vi "Teleop.vi"(10 "Match Info":T1={"Autonomous Elapsed Seconds"=0.0, "TeleOp Elapsed Seconds"=0.0, "Disabled Elapsed Seconds"=0.0, "Visited Autonomous"=FALSE, "Visited TeleOp"=FALSE, "Visited Disabled"=FALSE, "Autonomous Settings"={"Autonomous Style"=enum."Independent", "VI Refnum"=refnum}}, 11 "Call Context":T2) -> ()   [LabVIEW 2013]
doc: "This VI is called for each TeleOp packet received from the DS where the robot is not disabled. It is often used to read from the joysticks and update I/O or to update setpoints for timed control loops. It should complete and return within 20 milliseconds or it may miss DS packets."
uses:
  <vilib>/Rock Robotics/WPI/DriverStation/WPI_DriverStationDerivedRobotMode.ctl
  <vilib>/Rock Robotics/WPI/DriverStation/WPI_DriverStationMatch Info.ctl
  <vilib>/Rock Robotics/WPI/DriverStation/DriverStationLCD/WPI_DriverStationLCDLCDLine.ctl
  Robot Global Data.vi
  <vilib>/Rock Robotics/WPI/Joystick/WPI_JoystickGetSetRefNum.vi
  <vilib>/Rock Robotics/WPI/RobotDrive/WPI_RobotDriveGetSetRefNum.vi
  <vilib>/Rock Robotics/WPI/Solenoid/WPI_SolenoidSetEnum.vi
  <vilib>/Rock Robotics/WPI/Solenoid/WPI_SolenoidValue.ctl
panel:
  out "Numeric 1":dbl(slide) scale=0.0..100.0
  out "Boolean 2":bool
  out "Boolean 1":bool
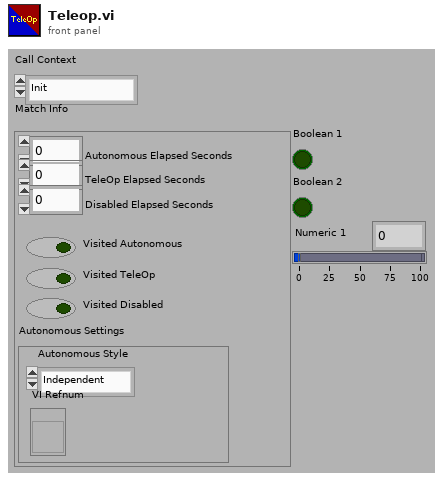
[diagram p1: front panel]
types:
  T1 = typedef "WPI_DriverStationMatch Info.ctl" = cluster{"Autonomous Elapsed Seconds":dbl, "TeleOp Elapsed Seconds":dbl, "Disabled Elapsed Seconds":dbl, "Visited Autonomous":bool, "Visited TeleOp":bool, "Visited Disabled":bool, "Autonomous Settings":cluster{"Autonomous Style":enum16{"Iterative", "Independent"}, "VI Refnum":refnum<vi>}}
  T2 = typedef "WPI_DriverStationDerivedRobotMode.ctl" = enum16{"Init", "Execute", "Stop"}
  T3 = typedef "WPI_DriverStationLCDLCDLine.ctl" = enum16{"Main - Line 1", "User - Line 2", "User - Line 3", "User - Line 4", "User - Line 5", "User - Line 6"}
  T4 = typedef "WPI_JoystickDevRef.ctl" = cluster{"Device":T5}
  T5 = typedef "WPI_JoystickDeviceEnum.ctl" = enum16{"USB 1", "USB 2", "USB 3", "USB 4", "Kinect 1", "Kinect 2"}
  T6 = typedef "WPI_JoystickButtonState.ctl" = cluster{"Button 1":bool, "Button 2":bool, "Button 3":bool, "Button 4":bool, "Button 5":bool, "Button 6":bool, "Button 7":bool, "Button 8":bool, "Button 9":bool, "Button 10":bool, "Button 11":bool, "Button 12":bool}
  T7 = cluster{"axis 1 (x)":dbl, "axis 2 (y)":dbl, "axis 3 (throttle)":dbl, "axis 4":dbl, "axis 5":dbl, "axis 6":dbl}
  T8 = typedef "WPI_SolenoidValue.ctl" = enum16{"Off", "On", "Forward", "Reverse"}
  T9 = typedef "WPI_SolenoidDevRef.ctl" = cluster{"DevStatus":errorcluster, "Solenoid Module":T10, "Forward Solenoid Channel":T11, "Reverse Solenoid Channel":T11}
  T10 = typedef "FPGA_TypedefSolenoidModule.ctl" = enum16{"Solenoid Module 1", "Solenoid Module 2"}
  T11 = typedef "WPI_SolenoidChannel.ctl" = enum8{"Solenoid 1", "Solenoid 2", "Solenoid 3", "Solenoid 4", "Solenoid 5", "Solenoid 6", "Solenoid 7", "Solenoid 8", "Invalid"}
  T12 = typedef "WPI_RobotDriveDevRef.ctl" = cluster{"DevStatus":errorcluster, "Motors[]":T13[], "Square Inputs":bool, "Max Output":dbl, "Isochronous":bool}
  T13 = typedef "WPI_MotorControlDeviceRef.ctl" = cluster{"DeviceStatus":errorcluster, "Type":enum16{"PWM", "CAN"}, "PWM":cluster{"Digital Module":T14, "PWM Channel":T15, "DeadBand":T16}, "CAN":cluster{"Device Number":u8, "Control Mode":T17, "Semaphore":T18, "Max Vout":dbl}, "Invert":bool, "TransformRef":T19, "InvTransformRef":T19}
  T14 = typedef "FPGA_TypedefDigitalModule.ctl" = enum16{"Digital Module 1", "Digital Module 2"}
  T15 = typedef "FPGA_DIOPWMChannel.ctl" = enum8{"PWM 1", "PWM 2", "PWM 3", "PWM 4", "PWM 5", "PWM 6", "PWM 7", "PWM 8", "PWM 9", "PWM 10", "Invalid"}
  T16 = typedef "WPI_PWMDeadband.ctl" = cluster{"Name":string, "maxPositivePwm":i32, "minPositivePwm":i32, "centerPwm":i32, "maxNegativePwm":i32, "minNegativePwm":i32, "angularRange":u16}
  T17 = typedef "WPI_CANJaguar_ControlMode.ctl" = enum8{"Percent VBus", "Current", "Speed", "Position", "Voltage"}
  T18 = typedef "Semaphore RefNum" = refnum<k1>
  T19 = typedef "WPI_PWMTransform_ConPane.ctl" = refnum<vi>
  T20 = enum16{"Reset", "Start", "Reset 2", "Manual", "Get ready to Fire", "Disengage Gearbox", "Ready to Fire", "Firing", "Firing Completed", "Reengage Gearbox"}
  T21 = typedef "WPI_DigitalInputDevRef.ctl" = cluster{"DevStatus":errorcluster, "DIO Channel":T22, "Digital Module":T14}
  T22 = typedef "FPGA_DIOChannel.ctl" = enum8{"DIO 1", "DIO 2", "DIO 3", "DIO 4", "DIO 5", "DIO 6", "DIO 7", "DIO 8", "DIO 9", "DIO 10", "DIO 11", "DIO 12", "DIO 13", "DIO 14", "Invalid"}
  T23 = typedef "WPI_AnalogChannelDevRef.ctl" = cluster{"DevStatus":errorcluster, "Analog Module":T24, "Analog Channel":T25}
  T24 = typedef "FPGA_TypedefAnalogModule.ctl" = enum16{"Analog Module 1", "Analog Module 2"}
  T25 = typedef "FPGA_AIChannel.ctl" = enum8{"AI 1", "AI 2", "AI 3", "AI 4", "AI 5", "AI 6", "AI 7", "AI 8", "Invalid"}
  T26 = typedef "WPI_RelayDevRef.ctl" = cluster{"DevStatus":errorcluster, "Relay Channel":T27, "Digital Module":T14, "Relay Direction":T28}
  T27 = typedef "FPGA_DIORelayChannel.ctl" = enum8{"Relay 1", "Relay 2", "Relay 3", "Relay 4", "Relay 5", "Relay 6", "Relay 7", "Relay 8", "Invalid"}
  T28 = typedef "WPI_RelayDirection.ctl" = enum16{"Both directions", "Forward only", "Reverse only"}
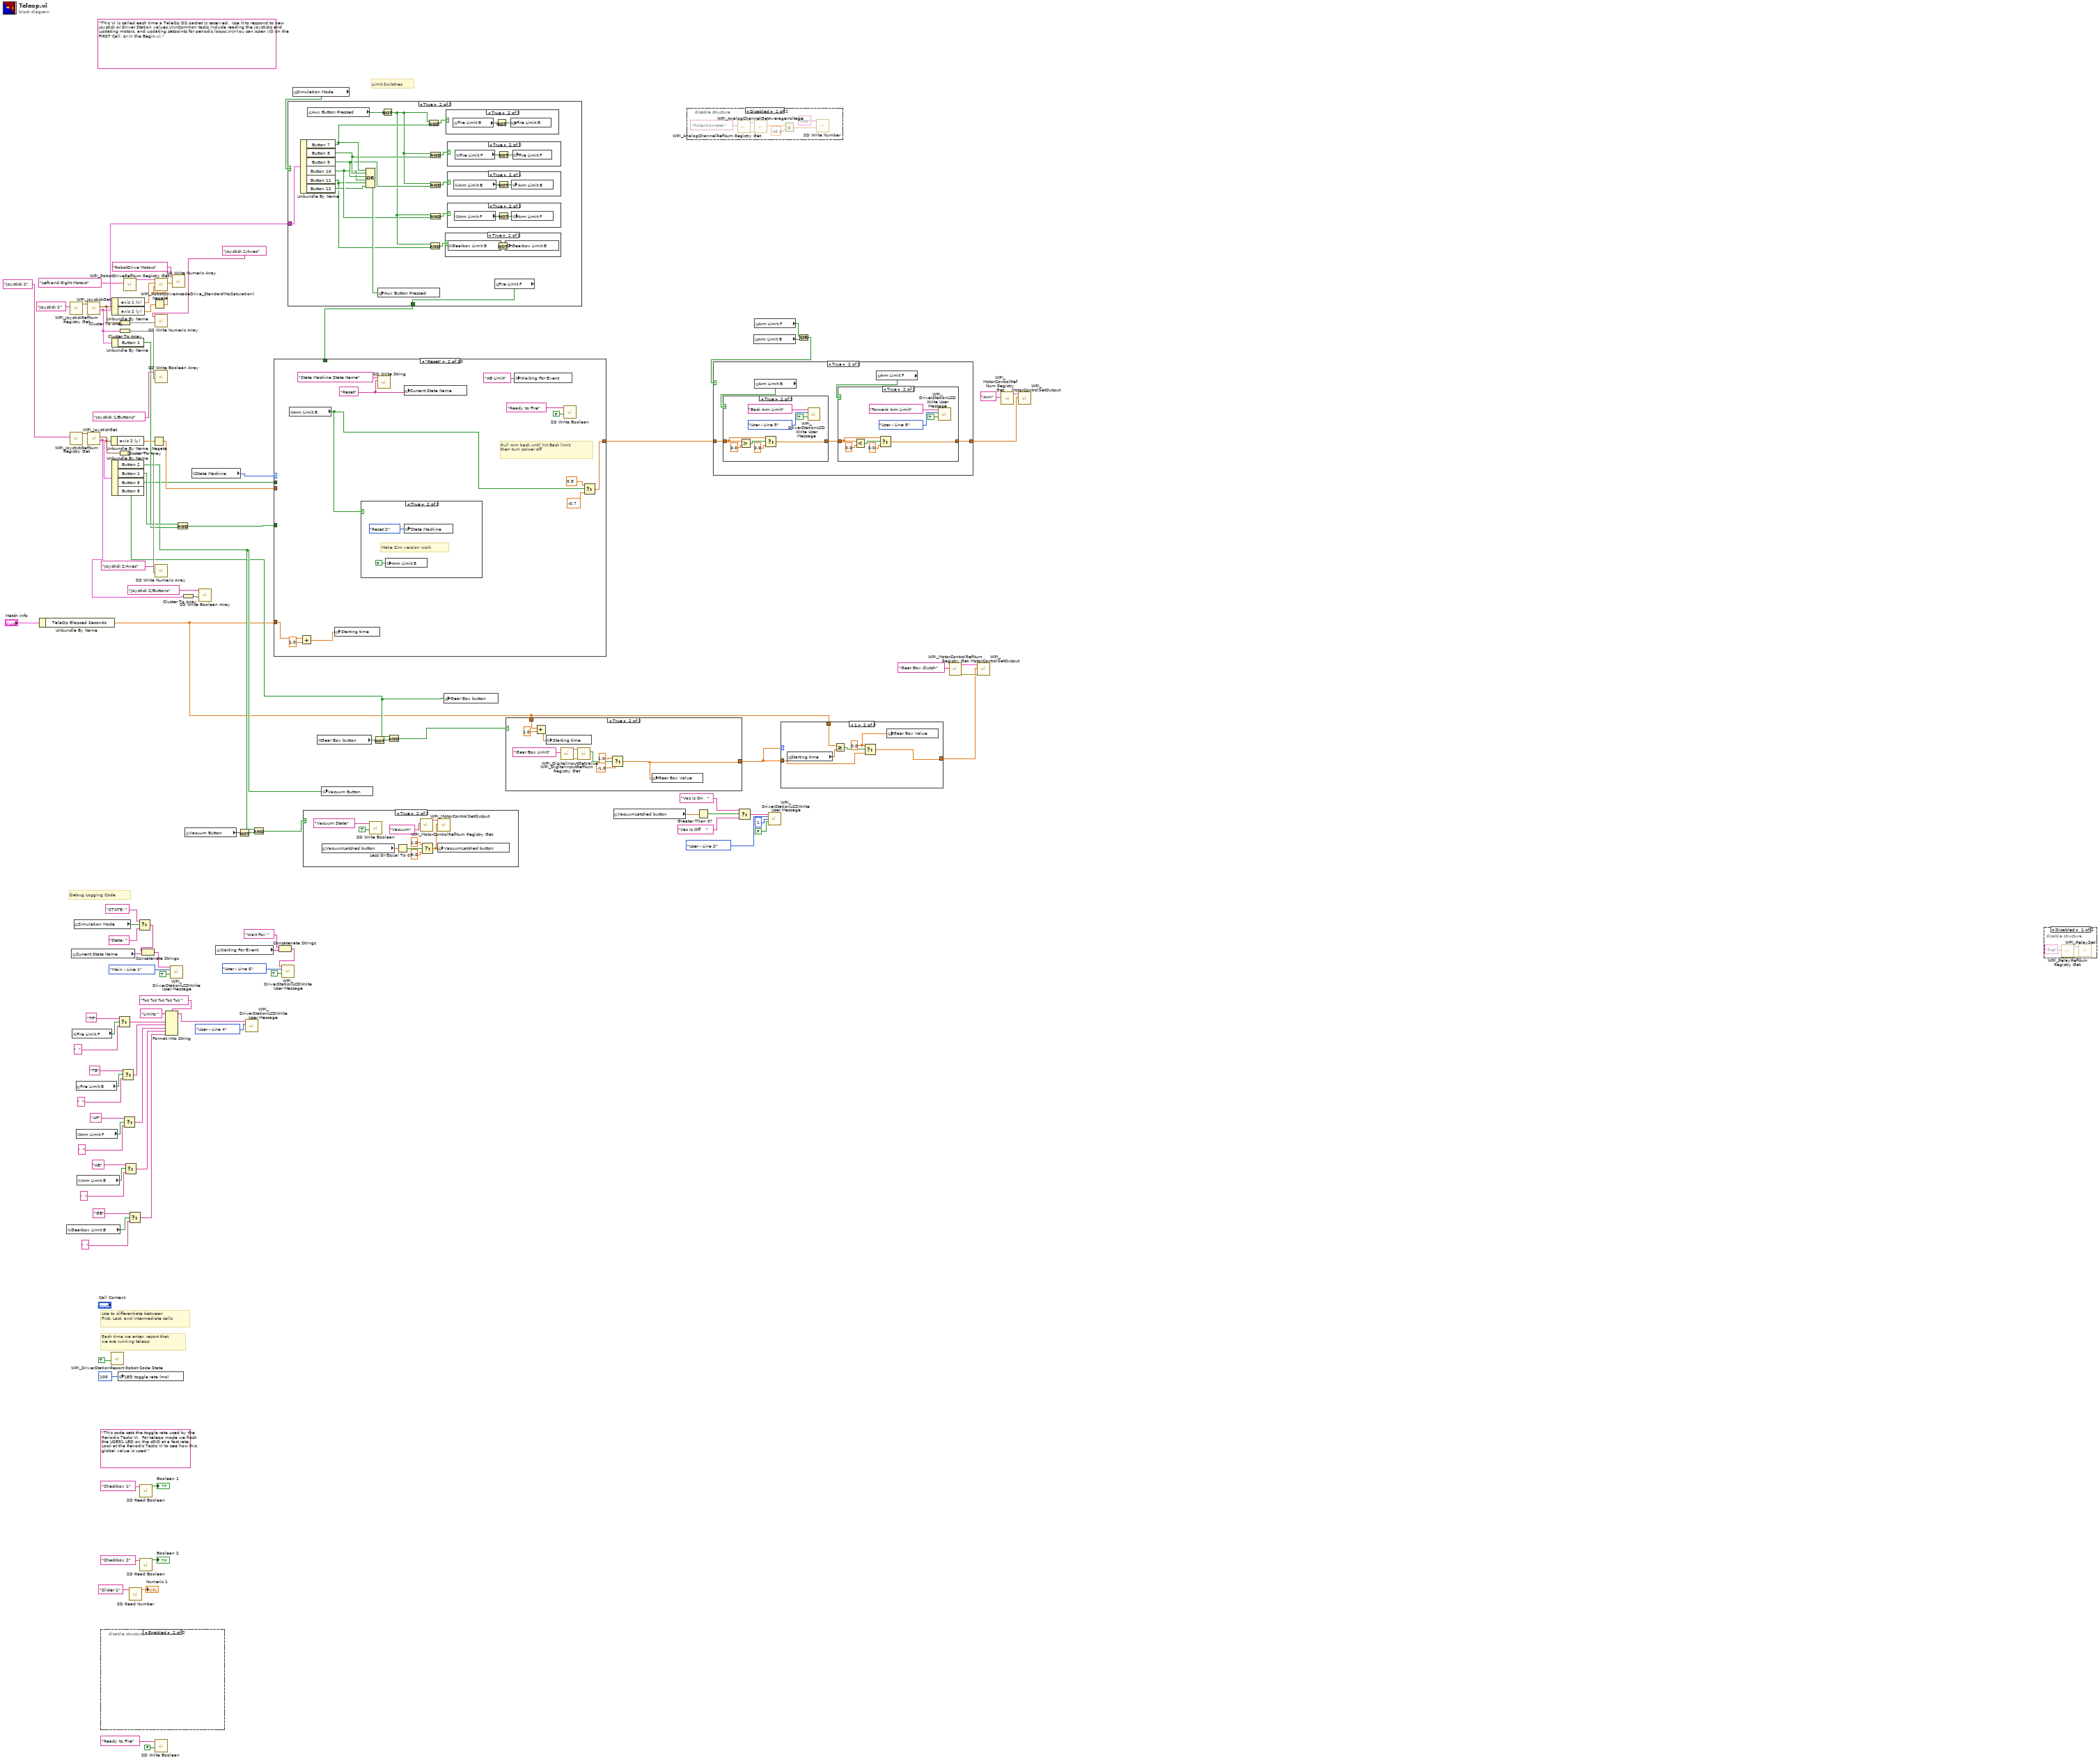
[diagram p0: block diagram]
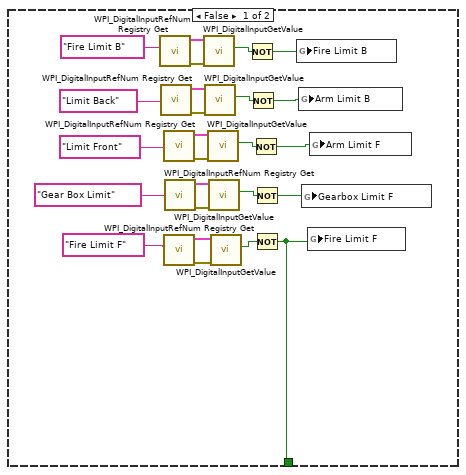
[diagram p2: hidden frame]
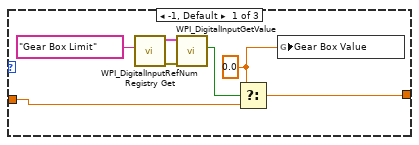
[diagram p8: hidden frame]
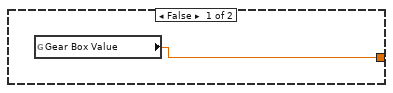
[diagram p10: hidden frame]
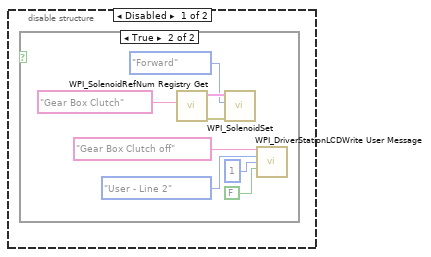
[diagram p17: hidden frame]
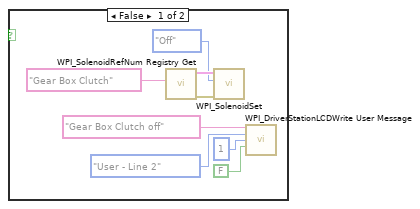
[diagram p18: hidden frame]
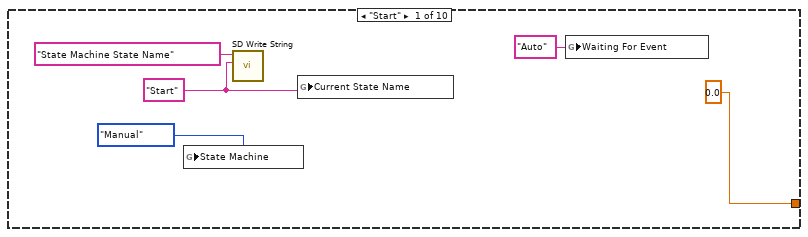
[diagram p19: hidden frame]
diagram:
  (unwired) "This code sets the toggle rate used by the Periodic Tasks VI.  For teleop mode we flash the USER1 LED on the cRIO at a fast rate.  Look at the Periodic Tasks VI to see how this global value is used."
  (unwired) "This VI is called each time a TeleOp DS packet is received.  Use it to respond to new joystick or Driver Station values.\n\nCommon tasks include reading the joysticks and updating motors, and updating setpoints for periodic loops.\n\nYou can open I/O on the FIRST Call, or in the Begin.vi."
  # "Limit Switches"
  # "Debug Logging Code"
  # "Each time we enter, report that\nwe are running teleop"
  # "Use to differentiate between\nFirst, Last, and Intermediate calls"
  n1 = Unbundle By Name("Match Info") -> ("TeleOp Elapsed Seconds"=w36:dbl)
  n2 = global read "Robot Global Data.vi" "Gearbox Limit B"() -> (w17:bool)
  n3 = call <vilib>:"WPI_JoystickRefNum Registry Get.vi"("refnum name"="Joystick 1") -> ("JoystickDevRef"=w104:T4)  [unwired: 1 in, 9 out]
  n4 = call <vilib>:"WPI_JoystickRefNum Registry Get.vi"("refnum name"="Joystick 2") -> ("JoystickDevRef"=w87:T4)  [unwired: 1 in, 9 out]
  n5 = global read "Robot Global Data.vi" "Current State Name"() -> (w52:string)
  n6 = global read "Robot Global Data.vi" "Fire Limit F"() -> (w21:bool)
  n7 = global read "Robot Global Data.vi" "Simulation Mode"() -> (w10:bool)
  n8 = global read "Robot Global Data.vi" "Fire Limit B"() -> (w20:bool)
  n9 = global read "Robot Global Data.vi" "Arm Limit F"() -> (w19:bool)
  n10 = global read "Robot Global Data.vi" "Arm Limit B"() -> (w18:bool)
  n11 = call <vilib>:"WPI_JoystickGet.vi"("JoystickDevRef"=w104) -> ("Buttons"=w6:T6, "Axes"=w99:T7)  [unwired: 1 in, 4 out]
  n12 = call <vilib>:"WPI_JoystickGet.vi"("JoystickDevRef"=w87) -> ("Buttons"=w81:T6, "Axes"=w84:T7)  [unwired: 1 in, 4 out]
  n13 = disable-structure shown="Enabled" {
    frame Disabled {
      n14 = case shown="True" {
        selector: _ -> [_ _]
        frame False {
          n15 = call <vilib>:"WPI_SolenoidRefNum Registry Get.vi"("refnum name"="Gear Box Clutch") -> ("error out"=w115:errorcluster, "SolenoidDevRef"=w116:T9)  [unwired: 9 in]
          n16 = call-poly <vilib>:"WPI_SolenoidSet.vi"("error in (no error)"=w115, "Value"=WPI_SolenoidValue."Off", "SolenoidDevRef"=w116) -> ()  [unwired: 7 in, 2 out]
          n17 = call <vilib>:"WPI_DriverStationLCDWrite User Message.vi"("line text"="Gear Box Clutch off", "line"=WPI_DriverStationLCDLCDLine."User - Line 2", "starting column"=i8 1, "clear line before write (T)"=FALSE) -> ()  [unwired: 11 in, 1 out]
        }
        frame True {
          n18 = call <vilib>:"WPI_SolenoidRefNum Registry Get.vi"("refnum name"="Gear Box Clutch") -> ("error out"=w123:errorcluster, "SolenoidDevRef"=w124:T9)  [unwired: 9 in]
          n19 = call-poly <vilib>:"WPI_SolenoidSet.vi"("error in (no error)"=w123, "Value"=WPI_SolenoidValue."Forward", "SolenoidDevRef"=w124) -> ()  [unwired: 7 in, 2 out]
          n20 = call <vilib>:"WPI_DriverStationLCDWrite User Message.vi"("line text"="Gear Box Clutch off", "line"=WPI_DriverStationLCDLCDLine."User - Line 2", "starting column"=i8 1, "clear line before write (T)"=FALSE) -> ()  [unwired: 11 in, 1 out]
        }
      }
    }
    frame Enabled {
    }
  }
  n21 = Unbundle By Name(w84) -> ("axis 2 (y)"=w80:dbl)
  n22 = call <vilib>:"WPI_DriverStationReport Robot Code State.vi"("TeleOp"=TRUE ("Autonomous")) -> ()  [unwired: 10 in, 1 out]
  n23 = Unbundle By Name(w99) -> ("axis 1 (x)"=w106:dbl, "axis 2 (y)"=w47:dbl)
  n24 = Unbundle By Name(w6) -> ("Button 1"=w78:bool)
  n25 = Unbundle By Name(w81) -> ("Button 2"=w69:bool, "Button 1"=w79:bool, "Button 5"=w55:bool, "Button 8"=w39:bool)
  n26 = Select(t="TF", s=w21, f="  ") -> (s? t:f=w27:string)
  n27 = global write "Robot Global Data.vi" "LED toggle rate (ms)"(u32 100 ("LED ms toggle rate")) -> ()
  n28 = Cluster To Array(cluster=w99) -> (array=w98:dbl[])
  n29 = Cluster To Array(cluster=w6) -> (array=w101:bool[])
  n30 = Cluster To Array(cluster=w84) -> (array=w83:dbl[])
  n31 = Select(t="TB", s=w20, f="  ") -> (s? t:f=w26:string)
  n32 = Select(t="AF", s=w19, f="  ") -> (s? t:f=w25:string)
  n33 = call <vilib>:"WPI_RobotDriveRefNum Registry Get.vi"("refnum name"="Left and Right Motors") -> ("RobotDriveDevRef"=w107:T12)  [unwired: 1 in, 9 out]
  n34 = Select(t="AB", s=w18, f="  ") -> (s? t:f=w24:string)
  n35 = Select(t="GB", s=w17, f="  ") -> (s? t:f=w23:string)
  n36 = call <vilib>:"SD Read Number.vi"("Name"="Slider 1" ("refnum name")) -> ("Numeric"=→"Numeric 1":dbl)  [unwired: 8 in, 2 out]
  n37 = Select(t="STATE: " ("line text"), s=w10, f="State: " ("line text")) -> (s? t:f=w7:string)
  n38 = call <vilib>:"SD Read Boolean.vi"("Name"="Checkbox 1" ("refnum name")) -> ("Boolean"=→"Boolean 1":bool)  [unwired: 8 in, 2 out]
  n39 = call <vilib>:"SD Read Boolean.vi"("Name"="Checkbox 2" ("refnum name")) -> ("Boolean"=→"Boolean 2":bool)  [unwired: 8 in, 2 out]
  n40 = Concatenate Strings(w7, w52) -> (w51:string)
  n41 = Negate(x=w80) -> (-x=w72:dbl)
  n42 = Negate(x=w47) -> (-x=w46:dbl)
  n43 = call <vilib>:"SD Write Boolean.vi"("Boolean"=FALSE, "Name"="Ready to Fire") -> ()  [unwired: 8 in, 2 out]
  n44 = call <vilib>:"WPI_RobotDriveArcadeDrive_Standard(NoSaturation).vi"("Y axis value"=w46, "X axis value"=w106, "RobotDriveDevRef"=w107) -> ("Motor Values"=w95:dbl[])  [unwired: 1 in, 7 out]
  n45 = call <vilib>:"SD Write Numeric Array.vi"("Numeric Array"=w98, "Name"="Joystick 1/Axes") -> ()  [unwired: 8 in, 2 out]
  n46 = call <vilib>:"SD Write Boolean Array.vi"("Boolean Array"=w101, "Name"="Joystick 1/Buttons") -> ()  [unwired: 8 in, 2 out]
  n47 = call <vilib>:"SD Write Numeric Array.vi"("Numeric Array"=w83, "Name"="Joystick 2/Axes") -> ()  [unwired: 8 in, 2 out]
  n48 = Format Into String(format string="%s %s %s %s %s " ("initial string"), initial string="Limits ", w27, w26, w25, w24, w23) -> (resulting string=w22:string)  [unwired: 1 in, 1 out]
  n49 = call <vilib>:"WPI_DriverStationLCDWrite User Message.vi"("line text"=w51, "line"=WPI_DriverStationLCDLCDLine."Main - Line 1", "clear line before write (T)"=TRUE) -> ()  [unwired: 12 in, 1 out]
  n50 = call <vilib>:"SD Write Numeric Array.vi"("Numeric Array"=w95, "Name"="RobotDrive Motors") -> ()  [unwired: 8 in, 2 out]
  n51 = And(x=w79, y=w78) -> (x .and. y?=w67:bool)
  n52 = Cluster To Array(cluster=w81) -> (array=w86:bool[])
  n53 = global read "Robot Global Data.vi" "Vacuum Button"() -> (w70:bool)
  n54 = global read "Robot Global Data.vi" "State Machine"() -> (w68:T20)
  n55 = call <vilib>:"SD Write Boolean Array.vi"("Boolean Array"=w86, "Name"="Joystick 2/Buttons") -> ()  [unwired: 8 in, 2 out]
  n56 = global read "Robot Global Data.vi" "Waiting For Event"() -> (w3:string)
  n57 = Not(x=w70) -> (.not. x?=w71:bool)
  n58 = call <vilib>:"WPI_DriverStationLCDWrite User Message.vi"("line text"=w22, "line"=WPI_DriverStationLCDLCDLine."User - Line 4") -> ()  [unwired: 13 in, 1 out]
  n59 = And(x=w69, y=w71) -> (x .and. y?=w65:bool)
  n60 = Concatenate Strings("Wait For: " ("string"), w3) -> (w1:string)
  n61 = call <vilib>:"WPI_DriverStationLCDWrite User Message.vi"("line text"=w1, "line"=WPI_DriverStationLCDLCDLine."User - Line 6", "clear line before write (T)"=TRUE) -> ()  [unwired: 12 in, 1 out]
  n62 = global read "Robot Global Data.vi" "Simulation Mode"() -> (w16:bool)
  n63 = case shown="True" w16 {
    tunnel: [w126 w154] -> w13
    tunnel: w6 -> [_ w166]
    frame False {
      n64 = call <vilib>:"WPI_DigitalInputRefNum Registry Get.vi"("refnum name"="Fire Limit B") -> ("error out"=w146:errorcluster, "DigitalInputDevRef"=w145:T21)  [unwired: 9 in]
      n65 = call <vilib>:"WPI_DigitalInputRefNum Registry Get.vi"("refnum name"="Limit Back") -> ("error out"=w142:errorcluster, "DigitalInputDevRef"=w141:T21)  [unwired: 9 in]
      n66 = call <vilib>:"WPI_DigitalInputRefNum Registry Get.vi"("refnum name"="Limit Front") -> ("error out"=w139:errorcluster, "DigitalInputDevRef"=w138:T21)  [unwired: 9 in]
      n67 = call <vilib>:"WPI_DigitalInputRefNum Registry Get.vi"("refnum name"="Fire Limit F") -> ("error out"=w149:errorcluster, "DigitalInputDevRef"=w150:T21)  [unwired: 9 in]
      n68 = call <vilib>:"WPI_DigitalInputRefNum Registry Get.vi"("refnum name"="Gear Box Limit") -> ("error out"=w135:errorcluster, "DigitalInputDevRef"=w134:T21)  [unwired: 9 in]
      n69 = call <vilib>:"WPI_DigitalInputGetValue.vi"("error in (no error)"=w146, "DigitalInputDevRef"=w145) -> ("Value"=w143:bool)  [unwired: 7 in, 2 out]
      n70 = call <vilib>:"WPI_DigitalInputGetValue.vi"("error in (no error)"=w142, "DigitalInputDevRef"=w141) -> ("Value"=w128:bool)  [unwired: 7 in, 2 out]
      n71 = call <vilib>:"WPI_DigitalInputGetValue.vi"("error in (no error)"=w139, "DigitalInputDevRef"=w138) -> ("Value"=w137:bool)  [unwired: 7 in, 2 out]
      n72 = call <vilib>:"WPI_DigitalInputGetValue.vi"("error in (no error)"=w135, "DigitalInputDevRef"=w134) -> ("Value"=w133:bool)  [unwired: 7 in, 2 out]
      n73 = call <vilib>:"WPI_DigitalInputGetValue.vi"("error in (no error)"=w149, "DigitalInputDevRef"=w150) -> ("Value"=w147:bool)  [unwired: 7 in, 2 out]
      n74 = Not(x=w143) -> (.not. x?=w127:bool)
      n75 = Not(x=w128) -> (.not. x?=w131:bool)
      n76 = Not(x=w137) -> (.not. x?=w130:bool)
      n77 = Not(x=w133) -> (.not. x?=w129:bool)
      n78 = Not(x=w147) -> (.not. x?=w126:bool)
      n79 = global write "Robot Global Data.vi" "Fire Limit B"(w127) -> ()
      n80 = global write "Robot Global Data.vi" "Arm Limit B"(w131) -> ()
      n81 = global write "Robot Global Data.vi" "Gearbox Limit F"(w129) -> ()
      n82 = global write "Robot Global Data.vi" "Fire Limit F"(w126) -> ()
      n83 = global write "Robot Global Data.vi" "Arm Limit F"(w130) -> ()
    }
    frame True {
      n84 = Unbundle By Name(w166) -> ("Button 7"=w164:bool, "Button 8"=w157:bool, "Button 9"=w156:bool, "Button 10"=w153:bool, "Button 11"=w151:bool, "Button 12"=w152:bool)
      n85 = global read "Robot Global Data.vi" "Aux Button Pressed"() -> (w165:bool)
      n86 = Compound Arithmetic op=OR(w164, w157, w156, w153, w151, w152) -> (w163:bool)
      n87 = global write "Robot Global Data.vi" "Aux Button Pressed"(w163) -> ()
      n88 = Not(x=w165) -> (.not. x?=w155:bool)
      n89 = And(x=w155, y=w164) -> (x .and. y?=w162:bool)
      n90 = And(x=w155, y=w151) -> (x .and. y?=w158:bool)
      n91 = And(x=w155, y=w157) -> (x .and. y?=w161:bool)
      n92 = And(x=w155, y=w156) -> (x .and. y?=w160:bool)
      n93 = And(x=w155, y=w153) -> (x .and. y?=w159:bool)
      n94 = case shown="True" w158 {
        frame False {
        }
        frame True {
          n95 = global read "Robot Global Data.vi" "Gearbox Limit B"() -> (w168:bool)
          n96 = Not(x=w168) -> (.not. x?=w167:bool)
          n97 = global write "Robot Global Data.vi" "Gearbox Limit B"(w167) -> ()
        }
      }
      n98 = case shown="True" w162 {
        frame False {
        }
        frame True {
          n99 = global read "Robot Global Data.vi" "Fire Limit B"() -> (w176:bool)
          n100 = Not(x=w176) -> (.not. x?=w175:bool)
          n101 = global write "Robot Global Data.vi" "Fire Limit B"(w175) -> ()
        }
      }
      n102 = case shown="True" w161 {
        frame False {
        }
        frame True {
          n103 = global read "Robot Global Data.vi" "Fire Limit F"() -> (w174:bool)
          n104 = Not(x=w174) -> (.not. x?=w173:bool)
          n105 = global write "Robot Global Data.vi" "Fire Limit F"(w173) -> ()
        }
      }
      n106 = case shown="True" w160 {
        frame False {
        }
        frame True {
          n107 = global read "Robot Global Data.vi" "Arm Limit B"() -> (w172:bool)
          n108 = Not(x=w172) -> (.not. x?=w171:bool)
          n109 = global write "Robot Global Data.vi" "Arm Limit B"(w171) -> ()
        }
      }
      n110 = case shown="True" w159 {
        frame False {
        }
        frame True {
          n111 = global read "Robot Global Data.vi" "Arm Limit F"() -> (w170:bool)
          n112 = Not(x=w170) -> (.not. x?=w169:bool)
          n113 = global write "Robot Global Data.vi" "Arm Limit F"(w169) -> ()
        }
      }
      n114 = global read "Robot Global Data.vi" "Fire Limit F"() -> (w154:bool)
    }
  }
  n115 = case shown="\"Reset\"" w68 {
    selector: w68 -> [_ _ w208 _ _ _ _ w275 _ _]
    tunnel: w72 -> [_ _ _ w219 _ w256 w267 w283 w293 w299]
    tunnel: [0.0 w189 0.0 w219 0.0 w256 w267 w283 w293 w299] -> w66
    tunnel: w67 -> [_ _ _ _ _ _ w263 _ _ _]
    tunnel: w36 -> [_ w186 w201 _ w236 w251 _ _ _ _]
    tunnel: w55 -> [_ _ _ w218 _ _ _ _ _ _]
    tunnel: w13 -> [_ _ _ _ _ _ _ _ _ _]
    frame "Start" {
      w179 = "Start" ("line text")
      n116 = global write "Robot Global Data.vi" "State Machine"(T20."Manual" ("State Machine")) -> ()
      n117 = call <vilib>:"SD Write String.vi"("Table Prefix"=w179, "Name"="State Machine State Name") -> ()  [unwired: 8 in, 2 out]
      n118 = global write "Robot Global Data.vi" "Current State Name"(w179) -> ()
      n119 = global write "Robot Global Data.vi" "Waiting For Event"("Auto" ("Waiting For Event")) -> ()
    }
    frame "Reset" {
      w187 = "Reset" ("line text")
      # "Pull Arm back until hit Back limit\nthen turn power off"
      n120 = global read "Robot Global Data.vi" "Arm Limit B"() -> (w182:bool)
      n121 = Add(x=w186, y=1.0) -> (x+y=w184:dbl)
      n122 = global write "Robot Global Data.vi" "Starting time"(w184) -> ()
      n123 = case shown="True" w182 {
        frame False {
        }
        frame True {
          # "Make Sim version work"
          n124 = global write "Robot Global Data.vi" "Arm Limit B"(FALSE ("Arm Limit B")) -> ()
          n125 = global write "Robot Global Data.vi" "State Machine"(T20."Reset 2" ("s? t:f")) -> ()
        }
      }
      n126 = call <vilib>:"SD Write String.vi"("Table Prefix"=w187, "Name"="State Machine State Name") -> ()  [unwired: 8 in, 2 out]
      n127 = global write "Robot Global Data.vi" "Current State Name"(w187) -> ()
      n128 = global write "Robot Global Data.vi" "Waiting For Event"("AB Limit" ("Waiting For Event")) -> ()
      n129 = call <vilib>:"SD Write Boolean.vi"("Boolean"=FALSE, "Name"="Ready to Fire") -> ()  [unwired: 8 in, 2 out]
      n130 = Select(t=0.5, s=w182, f=-0.7) -> (s? t:f=w189:dbl)
    }
    frame "Reset 2" {
      w203 = "Reset 2" ("line text")
      # "Reverse Trigger Motor until hit Back limit"
      n131 = global read "Robot Global Data.vi" "Starting time"() -> (w200:dbl)
      n132 = global read "Robot Global Data.vi" "Fire Limit B"() -> (w196:bool)
      n133 = Greater Or Equal?(x=w201, y=w200) -> (x >= y?=w199:bool)
      n134 = call <vilib>:"SD Write String.vi"("Table Prefix"=w203, "Name"="State Machine State Name") -> ()  [unwired: 8 in, 2 out]
      n135 = Or(x=w196, y=w199) -> (x .or. y?=w198:bool)
      n136 = global write "Robot Global Data.vi" "Current State Name"(w203) -> ()
      n137 = Select(t=T20."Manual" ("s? t:f"), s=w198, f=w208) -> (s? t:f=w207:T20)
      n138 = Select(t=0.0, s=w198, f=0.3) -> (s? t:f=w205:dbl)
      n139 = global write "Robot Global Data.vi" "State Machine"(w207) -> ()
      n140 = call <vilib>:"WPI_MotorControlRefNum Registry Get.vi"("refnum name"="Fire") -> ("error out"=w213:errorcluster, "MotorControlDevRef"=w212:T13)  [unwired: 9 in]
      n141 = call <vilib>:"WPI_MotorControlSetOutput.vi"("error in (no error)"=w213, "Output"=w205, "MotorControlDevRef"=w212) -> ()  [unwired: 6 in, 3 out]
      n142 = global write "Robot Global Data.vi" "Waiting For Event"("FB Limit" ("Waiting For Event")) -> ()
      n143 = call <vilib>:"SD Write Boolean.vi"("Boolean"=FALSE, "Name"="Ready to Fire") -> ()  [unwired: 8 in, 2 out]
    }
    frame "Manual", Default {
      w220 = "Manual" ("line text")
      # "If hit rear Arm limit switch, get ready to fire, \nelse if Reset button hit, start reset"
      n144 = global read "Robot Global Data.vi" "Arm Limit B"() -> (w217:bool)
      n145 = Or(x=w217, y=w218) -> (x .or. y?=w221:bool)
      n146 = case shown="True" w221 {
        tunnel: w217 -> [_ w230]
        frame False {
        }
        frame True {
          n147 = Select(t="Reason: Limit Back hit" ("line text"), s=w230, f="Reason Button 5 pressed:" ("line text")) -> (s? t:f=w225:string)
          n148 = Select(t=T20."Get ready to Fire" ("State Machine"), s=w230, f=T20."Reset" ("State Machine")) -> (s? t:f=w232:T20)
          n149 = global write "Robot Global Data.vi" "State Machine"(w232) -> ()
          n150 = call <vilib>:"WPI_DriverStationLCDWrite User Message.vi"("line text"=w225, "line"=WPI_DriverStationLCDLCDLine."User - Line 3", "clear line before write (T)"=TRUE) -> ()  [unwired: 12 in, 1 out]
        }
      }
      n151 = call <vilib>:"SD Write Boolean.vi"("Boolean"=FALSE, "Name"="Ready to Fire") -> ()  [unwired: 8 in, 2 out]
      n152 = call <vilib>:"SD Write String.vi"("Table Prefix"=w220, "Name"="State Machine State Name") -> ()  [unwired: 8 in, 2 out]
      n153 = global write "Robot Global Data.vi" "Current State Name"(w220) -> ()
      n154 = global write "Robot Global Data.vi" "Waiting For Event"("AB Limit | Btn 5" ("Waiting For Event")) -> ()
    }
    frame "Get ready to Fire" {
      w239 = "Get ready to Fire" ("line text")
      w245 = 0.0 ("f")
      # "Wait until hit gearbox limit switch"
      # "Disengage Gearbox"
      # "Turn Off Arm Motor"
      # "Turn Off Vacuum"
      n155 = global write "Robot Global Data.vi" "VacuumLatched button"(w245) -> ()
      n156 = Add(x=0.5 ("Starting time"), y=w236) -> (x+y=w237:dbl)
      n157 = call <vilib>:"WPI_MotorControlRefNum Registry Get.vi"("refnum name"="Vacuum") -> ("MotorControlDevRef"=w246:T13)  [unwired: 9 in, 1 out]
      n158 = global write "Robot Global Data.vi" "Starting time"(w237) -> ()
      n159 = call <vilib>:"WPI_MotorControlSetOutput.vi"("Output"=w245, "MotorControlDevRef"=w246) -> ()  [unwired: 7 in, 3 out]
      n160 = call <vilib>:"WPI_MotorControlRefNum Registry Get.vi"("refnum name"="Gear Box Clutch") -> ("MotorControlDevRef"=w244:T13)  [unwired: 9 in, 1 out]
      n161 = call <vilib>:"SD Write Boolean.vi"("Boolean"=TRUE, "Name"="Vacuum State") -> ()  [unwired: 8 in, 2 out]
      n162 = call <vilib>:"SD Write String.vi"("Table Prefix"=w239, "Name"="State Machine State Name") -> ()  [unwired: 8 in, 2 out]
      n163 = call <vilib>:"WPI_MotorControlSetOutput.vi"("Output"=1.0 ("Numeric"), "MotorControlDevRef"=w244) -> ()  [unwired: 7 in, 3 out]
      n164 = global write "Robot Global Data.vi" "Current State Name"(w239) -> ()
      n165 = global write "Robot Global Data.vi" "State Machine"(T20."Disengage Gearbox" ("State Machine")) -> ()
      n166 = global write "Robot Global Data.vi" "Waiting For Event"("Auto" ("Waiting For Event")) -> ()
    }
    frame "Disengage Gearbox" {
      w254 = "Disengage Gearbox" ("line text")
      # "When time completed, return to Manual control"
      n167 = global read "Robot Global Data.vi" "Starting time"() -> (w253:dbl)
      n168 = Greater Or Equal?(x=w251, y=w253) -> (x >= y?=w252:bool)
      n169 = call <vilib>:"SD Write String.vi"("Table Prefix"=w254, "Name"="State Machine State Name") -> ()  [unwired: 8 in, 2 out]
      n170 = case shown="True" w252 {
        frame False {
        }
        frame True {
          n171 = call <vilib>:"WPI_MotorControlRefNum Registry Get.vi"("refnum name"="Gear Box Clutch") -> ("MotorControlDevRef"=w260:T13)  [unwired: 9 in, 1 out]
          n172 = global write "Robot Global Data.vi" "State Machine"(T20."Ready to Fire" ("State Machine")) -> ()
          n173 = call <vilib>:"WPI_MotorControlSetOutput.vi"("Output"=0.0 ("Numeric"), "MotorControlDevRef"=w260) -> ()  [unwired: 7 in, 3 out]
        }
      }
      n174 = global write "Robot Global Data.vi" "Current State Name"(w254) -> ()
      n175 = global write "Robot Global Data.vi" "Waiting For Event"("Timer" ("Waiting For Event")) -> ()
    }
    frame "Ready to Fire" {
      w262 = "Ready to fire" ("line text")
      # "If both trigger btns pressed, fire"
      n176 = call <vilib>:"SD Write Boolean.vi"("Boolean"=FALSE, "Name"="Ready to Fire") -> ()  [unwired: 8 in, 2 out]
      n177 = call <vilib>:"SD Write String.vi"("Table Prefix"=w262, "Name"="State Machine State Name") -> ()  [unwired: 8 in, 2 out]
      n178 = global write "Robot Global Data.vi" "Current State Name"(w262) -> ()
      n179 = case shown="True" w263 {
        frame False {
        }
        frame True {
          n180 = global write "Robot Global Data.vi" "State Machine"(T20."Firing" ("State Machine")) -> ()
        }
      }
      n181 = global write "Robot Global Data.vi" "Waiting For Event"("Both Btn1s" ("Waiting For Event")) -> ()
    }
    frame "Firing" {
      w273 = "Firing" ("line text")
      # "Run Trigger motor forward until hit forward limit"
      n182 = global read "Robot Global Data.vi" "Fire Limit F"() -> (w269:bool)
      n183 = call <vilib>:"SD Write String.vi"("Table Prefix"=w273, "Name"="State Machine State Name") -> ()  [unwired: 8 in, 2 out]
      n184 = Select(t=T20."Firing Completed" ("s? t:f"), s=w269, f=w275) -> (s? t:f=w274:T20)
      n185 = global write "Robot Global Data.vi" "Current State Name"(w273) -> ()
      n186 = global write "Robot Global Data.vi" "State Machine"(w274) -> ()
      n187 = Select(t=0.0, s=w269, f=-0.8) -> (s? t:f=w277:dbl)
      n188 = call <vilib>:"WPI_MotorControlRefNum Registry Get.vi"("refnum name"="Fire") -> ("error out"=w282:errorcluster, "MotorControlDevRef"=w281:T13)  [unwired: 9 in]
      n189 = call <vilib>:"WPI_MotorControlSetOutput.vi"("error in (no error)"=w282, "Output"=w277, "MotorControlDevRef"=w281) -> ()  [unwired: 6 in, 3 out]
      n190 = global write "Robot Global Data.vi" "Waiting For Event"("FF Limit" ("Waiting For Event")) -> ()
      n191 = global write "Robot Global Data.vi" "Waiting For Event"("FF Limit" ("Waiting For Event")) -> ()
    }
    frame "Firing Completed" {
      w286 = "Firing Completed" ("line text")
      # "Run for .5 secs"
      # "Re-engage Gearbox by running clutch motor in reverse"
      # "Turn off Trigger motor"
      n192 = call <vilib>:"WPI_MotorControlRefNum Registry Get.vi"("refnum name"="Fire") -> ("error out"=w292:errorcluster, "MotorControlDevRef"=w291:T13)  [unwired: 9 in]
      n193 = call <vilib>:"WPI_MotorControlSetOutput.vi"("error in (no error)"=w292, "Output"=0.0, "MotorControlDevRef"=w291) -> ()  [unwired: 6 in, 3 out]
      n194 = call <vilib>:"SD Write String.vi"("Table Prefix"=w286, "Name"="State Machine State Name") -> ()  [unwired: 8 in, 2 out]
      n195 = global write "Robot Global Data.vi" "State Machine"(T20."Reengage Gearbox" ("State Machine")) -> ()
      n196 = global write "Robot Global Data.vi" "Gear Box Value"(-1.0 ("Numeric")) -> ()
      n197 = global write "Robot Global Data.vi" "Current State Name"(w286) -> ()
      n198 = global write "Robot Global Data.vi" "Waiting For Event"("Auto" ("Waiting For Event")) -> ()
    }
    frame "Reengage Gearbox" {
      w297 = "Reengage Gearbox" ("line text")
      # "Keep moving gearbox motor until hit limit switch"
      n199 = global read "Robot Global Data.vi" "Gearbox Limit B"() -> (w294:bool)
      n200 = global write "Robot Global Data.vi" "Waiting For Event"("GB Limit" ("Waiting For Event")) -> ()
      n201 = call <vilib>:"SD Write String.vi"("Table Prefix"=w297, "Name"="State Machine State Name") -> ()  [unwired: 8 in, 2 out]
      n202 = case shown="True" w294 {
        frame False {
        }
        frame True {
          n203 = global write "Robot Global Data.vi" "State Machine"(T20."Manual" ("State Machine")) -> ()
          n204 = call <vilib>:"WPI_MotorControlRefNum Registry Get.vi"("refnum name"="Gear Box Clutch") -> ("error out"=w300:errorcluster, "MotorControlDevRef"=w304:T13)  [unwired: 9 in]
          n205 = call <vilib>:"WPI_MotorControlSetOutput.vi"("error in (no error)"=w300, "Output"=0.0 ("Numeric"), "MotorControlDevRef"=w304) -> ()  [unwired: 6 in, 3 out]
        }
      }
      n206 = global write "Robot Global Data.vi" "Current State Name"(w297) -> ()
      n207 = global write "Robot Global Data.vi" "Waiting For Event"("GB Limit" ("Waiting For Event")) -> ()
    }
  }
  n208 = case shown="True" w65 {
    frame False {
    }
    frame True {
      n209 = global read "Robot Global Data.vi" "VacuumLatched button"() -> (w311:dbl)
      n210 = call <vilib>:"SD Write Boolean.vi"("Boolean"=TRUE, "Name"="Vacuum State") -> ()  [unwired: 8 in, 2 out]
      n211 = Less Or Equal To 0?(x=w311) -> (x <= 0?=w306:bool)
      n212 = call <vilib>:"WPI_MotorControlRefNum Registry Get.vi"("refnum name"="Vacuum") -> ("MotorControlDevRef"=w308:T13)  [unwired: 9 in, 1 out]
      n213 = Select(t=1.0 ("Numeric"), s=w306, f=0.0) -> (s? t:f=w307:dbl)
      n214 = call <vilib>:"WPI_MotorControlSetOutput.vi"("Output"=w307, "MotorControlDevRef"=w308) -> ()  [unwired: 7 in, 3 out]
      n215 = global write "Robot Global Data.vi" "VacuumLatched button"(w307) -> ()
    }
  }
  n216 = global read "Robot Global Data.vi" "Gear Box button"() -> (w41:bool)
  n217 = global write "Robot Global Data.vi" "Vacuum Button"(w69) -> ()
  n218 = Not(x=w41) -> (.not. x?=w42:bool)
  n219 = And(x=w39, y=w42) -> (x .and. y?=w40:bool)
  n220 = global write "Robot Global Data.vi" "Gear Box button"(w39) -> ()
  n221 = case shown="True" w40 {
    tunnel: w36 -> [_ w319]
    tunnel: [w314 w315] -> w37
    frame False {
      n222 = global read "Robot Global Data.vi" "Gear Box Value"() -> (w314:dbl)
    }
    frame True {
      n223 = Add(x=w319, y=1.0) -> (x+y=w323:dbl)
      n224 = global write "Robot Global Data.vi" "Starting time"(w323) -> ()
      n225 = call <vilib>:"WPI_DigitalInputRefNum Registry Get.vi"("refnum name"="Gear Box Limit") -> ("error out"=w321:errorcluster, "DigitalInputDevRef"=w322:T21)  [unwired: 9 in]
      n226 = call <vilib>:"WPI_DigitalInputGetValue.vi"("error in (no error)"=w321, "DigitalInputDevRef"=w322) -> ("Value"=w316:bool)  [unwired: 7 in, 2 out]
      n227 = Select(t=1.0, s=w316, f=-1.0) -> (s? t:f=w315:dbl)
      n228 = global write "Robot Global Data.vi" "Gear Box Value"(w315) -> ()
    }
  }
  n229 = global read "Robot Global Data.vi" "VacuumLatched button"() -> (w56:dbl)
  n230 = disable-structure shown="Disabled" {
    frame Disabled {
      n231 = call <vilib>:"WPI_AnalogChannelRefNum Registry Get.vi"("refnum name"="Potentiometer") -> ("error out"=w331:errorcluster, "AIDeviceRef"=w330:T23)  [unwired: 9 in]
      n232 = call <vilib>:"WPI_AnalogChannelGetAverageVoltage.vi"("error in (no error)"=w331, "AIDeviceRef"=w330) -> ("Voltage"=w326:dbl)  [unwired: 7 in, 2 out]
      n233 = Multiply(x=w326, y=45.0) -> (x*y=w325:dbl)
      n234 = call <vilib>:"SD Write Number.vi"("Numeric"=w325, "Name"="Pot") -> ()  [unwired: 8 in, 2 out]
    }
    frame Enabled {
    }
  }
  n235 = Greater Than 0?(x=w56) -> (x > 0?=w57:bool)
  n236 = Select(t="Vac Is On   ", s=w57, f="Vac Is Off    ") -> (s? t:f=w63:string)
  n237 = global read "Robot Global Data.vi" "Arm Limit B"() -> (w14:bool)
  n238 = global read "Robot Global Data.vi" "Arm Limit F"() -> (w15:bool)
  n239 = call <vilib>:"WPI_DriverStationLCDWrite User Message.vi"("line text"=w63, "line"=WPI_DriverStationLCDLCDLine."User - Line 2", "starting column"=i8 1, "clear line before write (T)"=FALSE) -> ()  [unwired: 11 in, 1 out]
  n240 = case shown="1" w37 {
    tunnel: [w334 w340 w345] -> w38
    tunnel: w37 -> [w333 w341 w345]
    tunnel: w36 -> [_ w344 _]
    frame -1, Default {
      w332 = 0.0 ("t")
      n241 = call <vilib>:"WPI_DigitalInputRefNum Registry Get.vi"("refnum name"="Gear Box Limit") -> ("error out"=w337:errorcluster, "DigitalInputDevRef"=w338:T21)  [unwired: 9 in]
      n242 = call <vilib>:"WPI_DigitalInputGetValue.vi"("error in (no error)"=w337, "DigitalInputDevRef"=w338) -> ("Value"=w335:bool)  [unwired: 7 in, 2 out]
      n243 = Select(t=w332, s=w335, f=w333) -> (s? t:f=w334:dbl)
      n244 = global write "Robot Global Data.vi" "Gear Box Value"(w332) -> ()
    }
    frame 1 {
      w339 = 0.0 ("t")
      n245 = global read "Robot Global Data.vi" "Starting time"() -> (w343:dbl)
      n246 = Greater Or Equal?(x=w344, y=w343) -> (x >= y?=w342:bool)
      n247 = Select(t=w339, s=w342, f=w341) -> (s? t:f=w340:dbl)
      n248 = global write "Robot Global Data.vi" "Gear Box Value"(w339) -> ()
    }
    frame 0 {
    }
  }
  n249 = Or(x=w15, y=w14) -> (x .or. y?=w73:bool)
  n250 = case shown="True" w73 {
    tunnel: w66 -> [w346 w351]
    tunnel: [w346 w349] -> w64
    frame False {
    }
    frame True {
      n251 = global read "Robot Global Data.vi" "Arm Limit B"() -> (w348:bool)
      n252 = case shown="True" w348 {
        tunnel: w351 -> [w361 w367]
        tunnel: [w361 w369] -> w350
        frame False {
        }
        frame True {
          n253 = Greater?(x=w367, y=0.0) -> (0:w365:bool)
          n254 = Select(t=w367, s=w365, f=0.0) -> (s? t:f=w369:dbl)
          n255 = call <vilib>:"WPI_DriverStationLCDWrite User Message.vi"("line text"="Back Arm Limit", "line"=WPI_DriverStationLCDLCDLine."User - Line 5", "clear line before write (T)"=TRUE) -> ()  [unwired: 12 in, 1 out]
        }
      }
      n256 = global read "Robot Global Data.vi" "Arm Limit F"() -> (w347:bool)
      n257 = case shown="True" w347 {
        tunnel: w350 -> [w352 w358]
        tunnel: [w352 w360] -> w349
        frame False {
        }
        frame True {
          n258 = Less?(x=w358, y=0.0) -> (x < y?=w356:bool)
          n259 = Select(t=w358, s=w356, f=0.0) -> (s? t:f=w360:dbl)
          n260 = call <vilib>:"WPI_DriverStationLCDWrite User Message.vi"("line text"="Forward Arm Limit", "line"=WPI_DriverStationLCDLCDLine."User - Line 5", "clear line before write (T)"=TRUE) -> ()  [unwired: 12 in, 1 out]
        }
      }
    }
  }
  n261 = call <vilib>:"WPI_MotorControlRefNum Registry Get.vi"("refnum name"="Gear Box Clutch") -> ("error out"=w45:errorcluster, "MotorControlDevRef"=w43:T13)  [unwired: 9 in]
  n262 = call <vilib>:"WPI_MotorControlSetOutput.vi"("error in (no error)"=w45, "Output"=w38, "MotorControlDevRef"=w43) -> ()  [unwired: 6 in, 3 out]
  n263 = call <vilib>:"WPI_MotorControlRefNum Registry Get.vi"("refnum name"="Arm") -> ("MotorControlDevRef"=w75:T13)  [unwired: 9 in, 1 out]
  n264 = call <vilib>:"WPI_MotorControlSetOutput.vi"("Output"=w64, "MotorControlDevRef"=w75) -> ()  [unwired: 7 in, 3 out]
  n265 = disable-structure shown="Disabled" {
    frame Disabled {
      n266 = call <vilib>:"WPI_RelayRefNum Registry Get.vi"("refnum name"="fire") -> ("error out"=w371:errorcluster, "RelayDevRef"=w372:T26)  [unwired: 9 in]
      n267 = call <vilib>:"WPI_RelaySet.vi"("error in (no error)"=w371, "RelayDevRef"=w372) -> ()  [unwired: 8 in, 2 out]
    }
    frame Enabled {
    }
  }
